vi "External Pwr Ctrl Messenger.vi"(0 "Notifier Name":string, 2 "Actions":T1, 5 "Wavelength":string, 7 "Line On/Off":bool, 9 "Power (%)":dbl, 13 "Control Parameters":variant) -> ()   [LabVIEW 2020]
uses:
  External Power Control Type Defs/External Power Actions.ctl
  External Power Control Type Defs/External Power Notifier Type.ctl
panel:
  out "Error Out":errorcluster
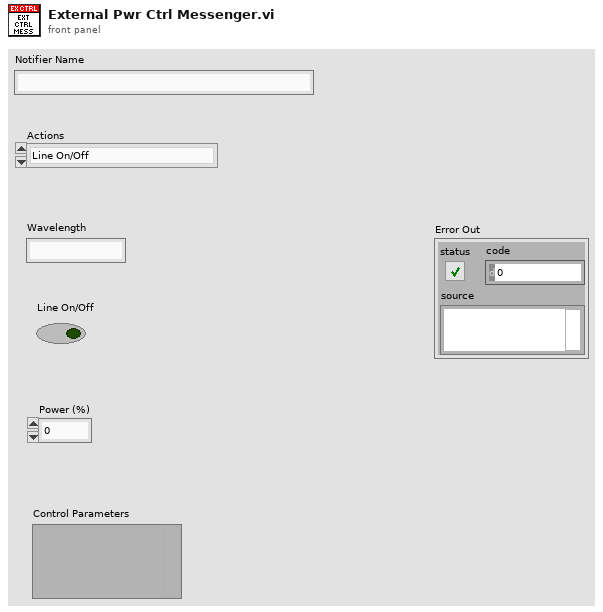
[diagram p1: front panel]
types:
  T1 = typedef "External Power Actions.ctl" = enum16{"Line On/Off", "Set Power", "Set Ctrl Parameters", "Quit"}
  T2 = typedef "External Power Notifier Type.ctl" = cluster{"Actions":T1, "Wavelength":string, "Line On/Off":bool, "Power (%)":dbl, "Control Parameters":variant, "Cmd Done?":bool}
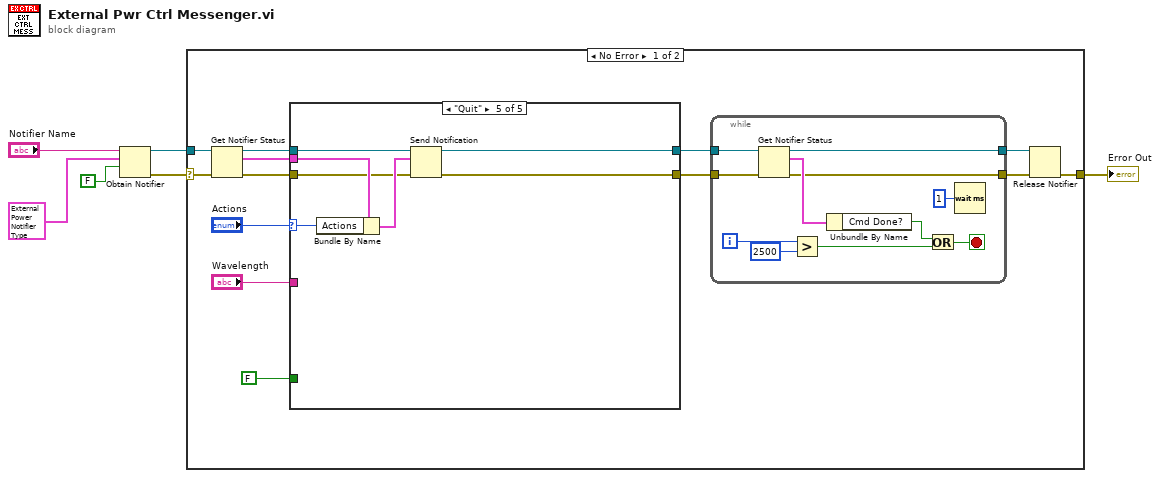
[diagram p0: block diagram]
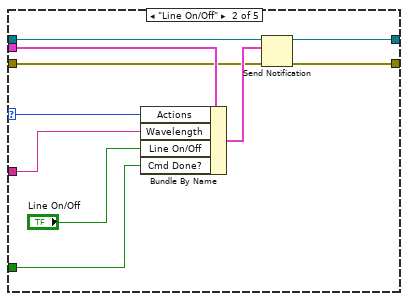
[diagram p3: hidden frame]
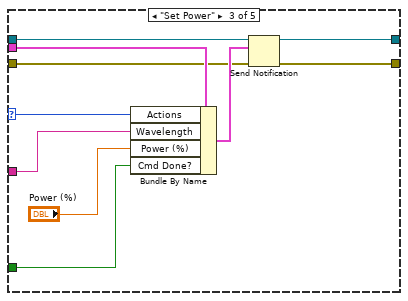
[diagram p4: hidden frame]
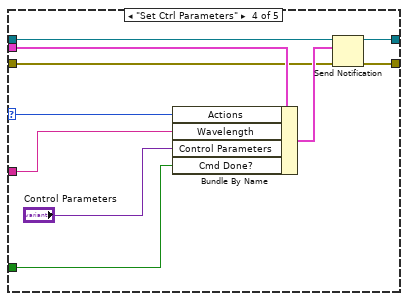
[diagram p5: hidden frame]
diagram:
  n1 = Obtain Notifier(name (unnamed)="Notifier Name", notification data type=T2 {"Actions"=enum."Line On/Off", "Wavelength"="", "Line On/Off"=FALSE, "Power (%)"=0.0, "Control Parameters"=variant, "Cmd Done?"=FALSE} ("External Ctrl"), create if not found? (T)=FALSE) -> (notifier out=w2:refnum<notifier>, error out=w3:errorcluster)  [unwired: 1 in, 1 out]
  n2 = case shown="No Error" w3 {
    selector: w3 -> [w17 w70]
    tunnel: w2 -> [w18 _]
    tunnel: [w7 w70] -> w1
    frame No Error {
      n3 = Get Notifier Status(notifier=w18, error in (no error)=w17) -> (notifier out=w16:refnum<notifier>, current notification=w15:T2, error out=w10:errorcluster)  [unwired: 2 out]
      n4 = case shown="\"Quit\"" "Actions" {
        selector: "Actions" -> [_ w41 w51 w61 w68]
        tunnel: w16 -> [w32 w38 w49 w59 w67]
        tunnel: w15 -> [_ w42 w52 w62 w69]
        tunnel: "Wavelength" -> [_ w40 w50 w60 _]
        tunnel: [w32 w36 w47 w57 w65] -> w12
        tunnel: FALSE -> [_ w35 w45 w55 _]
        tunnel: w10 -> [w31 w34 w44 w54 w64]
        tunnel: [w31 w33 w43 w53 w63] -> w9
        frame Default {
        }
        frame "Line On/Off" {
          n5 = Bundle By Name(cluster=w42, "Actions"=w41, "Wavelength"=w40, "Line On/Off"="Line On/Off", "Cmd Done?"=w35) -> (w37:T2)
          n6 = Send Notification(notification=w37, notifier=w38, error in (no error)=w34) -> (notifier out=w36:refnum<notifier>, error out=w33:errorcluster)
        }
        frame "Set Power" {
          n7 = Bundle By Name(cluster=w52, "Actions"=w51, "Wavelength"=w50, "Power (%)"="Power (%)", "Cmd Done?"=w45) -> (w48:T2)
          n8 = Send Notification(notification=w48, notifier=w49, error in (no error)=w44) -> (notifier out=w47:refnum<notifier>, error out=w43:errorcluster)
        }
        frame "Set Ctrl Parameters" {
          n9 = Bundle By Name(cluster=w62, "Actions"=w61, "Wavelength"=w60, "Control Parameters"="Control Parameters", "Cmd Done?"=w55) -> (w58:T2)
          n10 = Send Notification(notification=w58, notifier=w59, error in (no error)=w54) -> (notifier out=w57:refnum<notifier>, error out=w53:errorcluster)
        }
        frame "Quit" {
          n11 = Bundle By Name(cluster=w69, "Actions"=w68) -> (w66:T2)
          n12 = Send Notification(notification=w66, notifier=w67, error in (no error)=w64) -> (notifier out=w65:refnum<notifier>, error out=w63:errorcluster)
        }
      }
      n13 = while {
        tunnel: w12 -> [w30]
        tunnel: [w29] -> w11
        tunnel: w9 -> [w21]
        tunnel: [w20] -> w8
        i -> [w26]
        stop <- w22 stop-if-true
        n14 = Get Notifier Status(notifier=w30, error in (no error)=w21) -> (notifier out=w29:refnum<notifier>, current notification=w28:T2, error out=w20:errorcluster)  [unwired: 2 out]
        n15 = Greater?(x=w26, y=2500) -> (0:w24:bool)
        n16 = Unbundle By Name(w28) -> ("Cmd Done?"=w23:bool)
        n17 = Or(x=w23, y=w24) -> (x .or. y?=w22:bool)
        n18 = Wait (ms)(milliseconds to wait=u32 1) -> ()  [unwired: 1 out]
      }
      n19 = Release Notifier(notifier=w11, error in (no error)=w8) -> (error out=w7:errorcluster)  [unwired: 1 in, 2 out]
    }
    frame Error {
    }
  }
  "Error Out" <- w1
